vi "SafeSend.vi"(10 "EventAckn":bool, 11 "Event":bool) -> (3 "Boolean 3":bool)   [LabVIEW 2017]
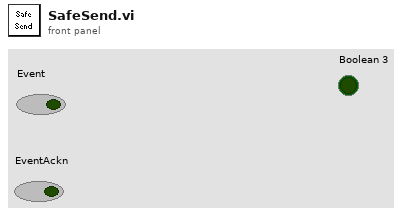
[diagram p1: front panel]
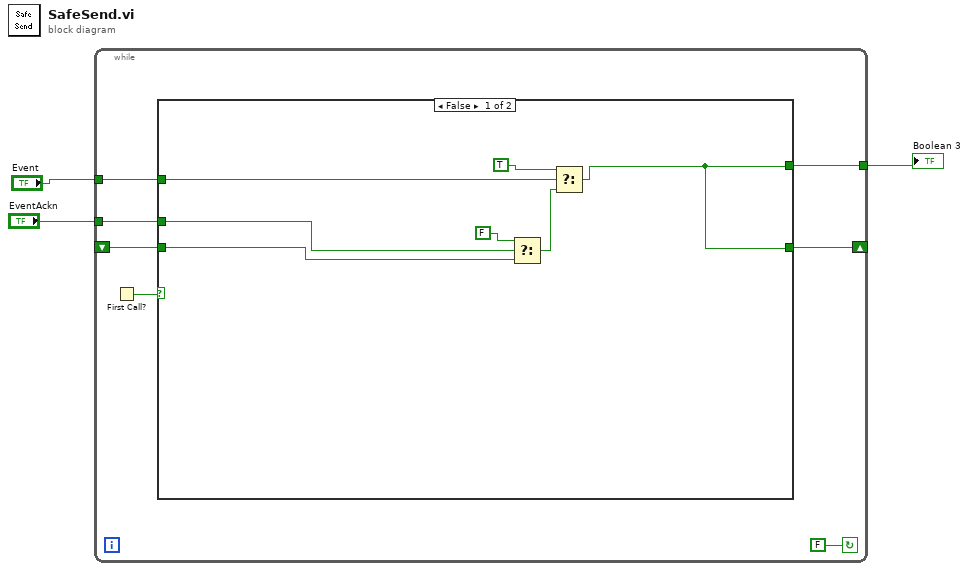
[diagram p0: block diagram]
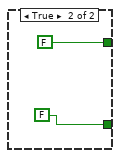
[diagram p2: hidden frame]
diagram:
  n1 = while {
    tunnel: [w8] -> w3
    shift-right: [w7] -> _
    shift-left: _ -> [w4]
    tunnel: "Event" -> [w6]
    tunnel: "EventAckn" -> [w5]
    stop <- FALSE continue-if-true
    n2 = First Call?() -> (First Call?: T/F=w9:bool)
    n3 = case shown="False" w9 {
      tunnel: [w11 FALSE ("Boolean 3")] -> w8
      tunnel: [w11 FALSE ("Boolean 3")] -> w7
      tunnel: w6 -> [w16 _]
      tunnel: w5 -> [w13 _]
      tunnel: w4 -> [w12 _]
      frame False {
        n4 = Select(t=FALSE, s=w13, f=w12) -> (s? t:f=w14:bool)
        n5 = Select(t=TRUE, s=w16, f=w14) -> (s? t:f=w11:bool)
      }
      frame True {
      }
    }
  }
  "Boolean 3" <- w3
